vi "Define Action.vi"(8 "Error In":errorcluster, 9 "Measurement":refnum<class "IAction.lvclass">, 10 "Name":string, 11 "Logger In":refnum<class "LoggerAPI.lvclass">) -> (0 "Error Out":errorcluster, 3 "Logger Out":refnum<class "LoggerAPI.lvclass">)   [LabVIEW 2020, in "LoggerAPI.lvclass"]
uses:
  LoggerAPI.lvclass
  IAction/IAction.lvclass
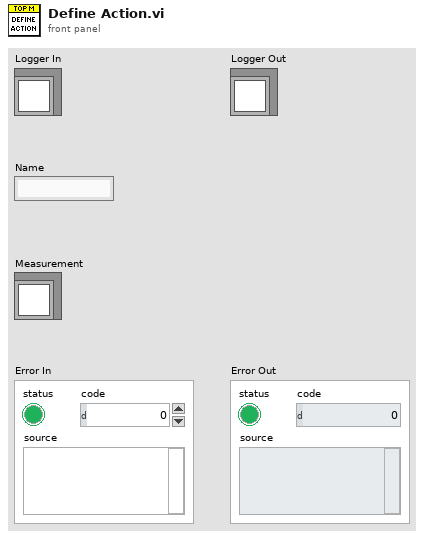
[diagram p1: front panel]
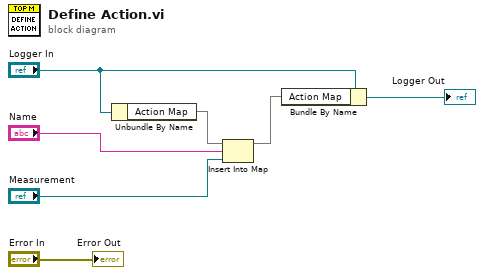
[diagram p0: block diagram]
diagram:
  n1 = Unbundle By Name("Logger In") -> ("Action Map"=w5:map{string, refnum<class "IAction.lvclass">})
  n2 = Insert Into Map(map in=w5, key="Name", value="Measurement") -> (map out=w6:map{string, refnum<class "IAction.lvclass">})  [unwired: 2 out]
  n3 = Bundle By Name(cluster="Logger In", "Action Map"=w6) -> (→"Logger Out":refnum<class "LoggerAPI.lvclass">)
  "Error Out" <- "Error In"
